vi "MOCKBEAR_Meter_to_Frequency.vi"(8 "error in (no error)":errorcluster, 10 "Meter":dbl format="%#_13g", 11 "MOCKBEAR in":refnum<class "MOCKBEAR.lvclass">) -> (0 "error out":errorcluster, 2 "Frequency":dbl, 3 "MOCKBEAR out":refnum<class "MOCKBEAR.lvclass">)   [LabVIEW 2021, in "MOCKBEAR.lvclass"]
uses:
  MOCKBEAR.lvclass
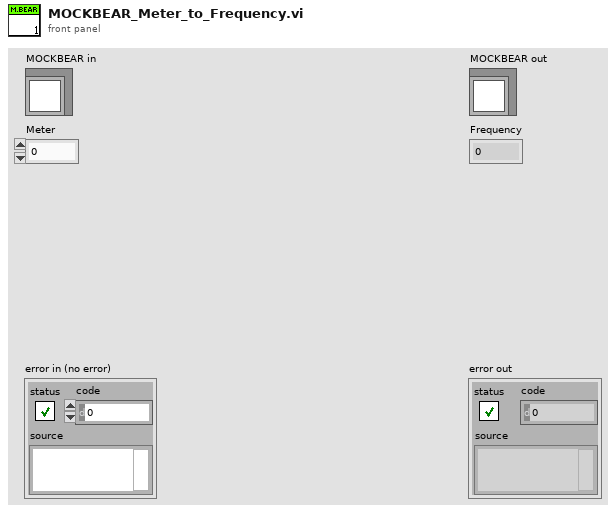
[diagram p1: front panel]
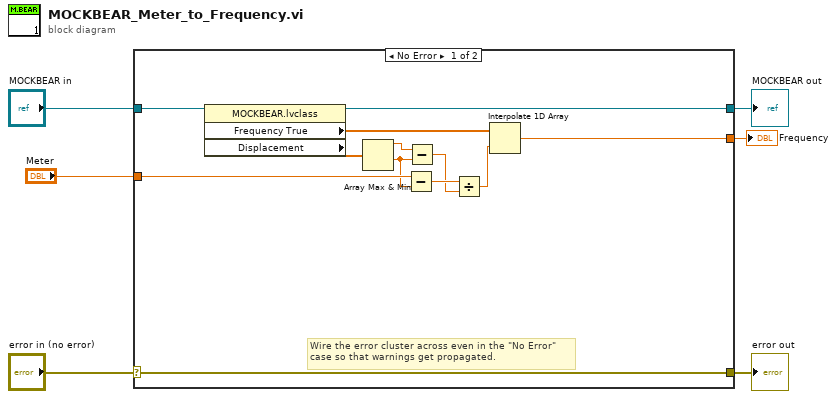
[diagram p0: block diagram]
diagram:
  n1 = case shown="No Error" "error in (no error)" {
    selector: "error in (no error)" -> [w18 w20]
    tunnel: [w18 w20] -> w5
    tunnel: [w7 w19] -> w3
    tunnel: "MOCKBEAR in" -> [w17 w19]
    tunnel: "Meter" -> [w15 _]
    tunnel: [w8 _] -> w1
    frame No Error {
      # "Wire the error cluster across even in the \"No Error\"\ncase so that warnings get propagated."
      n2 = property class="MOCKBEAR.lvclass"(reference=w17) -> (reference out=w7:refnum<class "MOCKBEAR.lvclass">, "Frequency True"=w10:dbl[], "Displacement"=w16:dbl[])  [unwired: 1 in, 1 out]
      n3 = Array Max & Min(array=w16) -> (max value=w14:dbl, min value=w13:dbl)  [unwired: 2 out]
      n4 = Subtract(x=w15, y=w13) -> (x-y=w12:dbl)
      n5 = Subtract(x=w14, y=w13) -> (x-y=w11:dbl)
      n6 = Divide(x=w12, y=w11) -> (x/y=w9:dbl)
      n7 = Interpolate 1D Array(1:w9, 2:w10) -> (0:w8:dbl)
    }
    frame Error {
    }
  }
  "error out" <- w5
  "MOCKBEAR out" <- w3
  "Frequency" <- w1
